vi "Calculate ENBW Butterworth.vi"(10 "time constant (s)":dbl, 11 "filter order":i32) -> (3 "ENBW (Hz)":dbl)   [LabVIEW 2019, in "DSP.lvclass"]
uses:
  DSP.lvclass
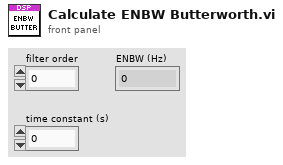
[diagram p1: front panel]
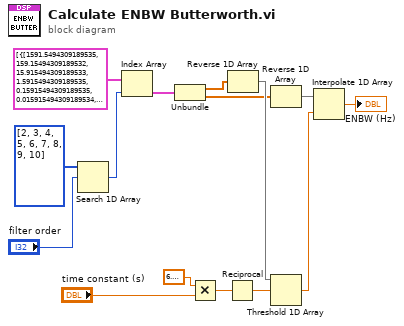
[diagram p0: block diagram]
diagram:
  n1 = Search 1D Array(1D array=i32[] [2, 3, 4, 5, 6, 7, 8, 9, 10] ("Array"), element="filter order") -> (index of element=w4:i32)  [unwired: 1 in]
  n2 = Index Array(array=cluster{dbl[], dbl[]}[] [{[1591.5494309189535, 159.15494309189532, 15.915494309189533, 1.5915494309189535, 0.15915494309189535, 0.015915494309189534, 0.0015915494309189533], [1767.099740912122, 176.77509646524533, 17.676678810580086, 1.7667678894862797, 0.17577664872265833, 0.016638452343507144, 0.0008956632431088917]}, {[1591.5494309189535, 159.15494309189532, 15.915494309189533, 1.5915494309189535, 0.15915494309189535, 0.015915494309189534, 0.0015915494309189533], [1666.5013949938002, 166.66559537189198, 16.66567589334608, 1.6656672905453724, 0.16566590855865096, 0.015640711483454667, 0.0007115391462718495]}, {[1591.5494309189535, 159.15494309189532, 15.915494309189533, 1.5915494309189535, 0.15915494309189535, 0.015915494309189534, 0.0015915494309189533], [1633.1249729596805, 163.31938425094248, 16.331046152781898, 1.6322040848298347, 0.16231834334347942, 0.015273471245026421, 0.0006415507485982914]}, {[1591.5494309189535, 159.15494309189532, 15.915494309189533, 1.5915494309189535, 0.15915494309189535, 0.015915494309189534, 0.0015915494309189533], [1617.9870361484807, 161.80244348926595, 16.17934893355119, 1.6170344814424644, 0.1608011553281375, 0.015126362044504297, 0.0005597638020751991]}, {[1591.5494309189535, 159.15494309189532, 15.915494309189533, 1.5915494309189535, 0.15915494309189535, 0.015915494309189534, 0.0015915494309189533], [1609.8449378687549, 160.98669739729402, 16.09777278146849, 1.608876591490976, 0.15998427250574704, 0.01501341797724548, 0.0005410281358335853]}, {[1591.5494309189535, 159.15494309189532, 15.915494309189533, 1.5915494309189535, 0.15915494309189535, 0.015915494309189534, 0.0015915494309189533], [1604.9628114166244, 160.49761135922873, 16.04886327886417, 1.6039855779052405, 0.1594937978511623, 0.014979592854989706, 0.000488757868653753]}, {[1591.5494309189535, 159.15494309189532, 15.915494309189533, 1.5915494309189535, 0.15915494309189535, 0.015915494309189534, 0.0015915494309189533], [1601.8050566605493, 160.18128906323892, 16.017230494249855, 1.6008223170852807, 0.1591757267331502, 0.014916206222619148, 0.0004311266700662223]}, {[1591.5494309189535, 159.15494309189532, 15.915494309189533, 1.5915494309189535, 0.15915494309189535, 0.015915494309189534, 0.0015915494309189533], [1599.6450662690663, 159.96492391147012, 15.9955936144505, 1.598658482860332, 0.15895977041310844, 0.014913270116707266, 0.00044571712858833496]}, {[1591.5494309189535, 159.15494309189532, 15.915494309189533, 1.5915494309189535, 0.15915494309189535, 0.015915494309189534, 0.0015915494309189533], [1598.102505316461, 159.81041021148107, 15.980141944847217, 1.5971131797141296, 0.15880336850266868, 0.014867311942267088, 0.00045600528696067044]}] ("XY Graph 6"), index=w4) -> (element=w8:cluster{dbl[], dbl[]})
  n3 = Unbundle(w8) -> (w9:dbl[], w11:dbl[])
  n4 = Multiply(x=6.283185307179586, y="time constant (s)") -> (x*y=w7:dbl)
  n5 = Reciprocal(x=w7) -> (1/x=w10:dbl)
  n6 = Reverse 1D Array(array=w9) -> (reversed array=w14:dbl[])
  n7 = Reverse 1D Array(array=w11) -> (reversed array=w15:dbl[])
  n8 = Threshold 1D Array(2:w10, 3:w14) -> (0:w12:dbl)  [unwired: 1 in]
  n9 = Interpolate 1D Array(1:w12, 2:w15) -> (0:→"ENBW (Hz)":dbl)
